vi "Write Ext.vi"(8 "Error In":errorcluster) -> (0 "Error Out":errorcluster)   [LabVIEW 2017, in "Tests.lvlib" / "Writer.lvlib"]
uses:
  Writer.lvlib
  src/LabPack/Public/Writer/Private/Write Ext by Value.vi
  <vilib>/addons/_JKI Toolkits/Caraya/classes/Test/Test.lvclass
  <vilib>/addons/_JKI Toolkits/Caraya/classes/Assert/Assert.lvclass
  src/LabPack/Public/Writer/Writer.lvclass
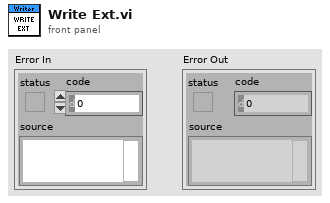
[diagram p1: front panel]
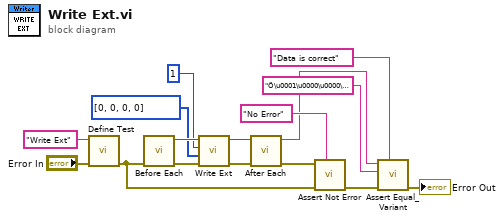
[diagram p0: block diagram]
diagram:
  n1 = call <vilib>:"Define Test.vi"("error in (no error)"="Error In", "Label (VI Title)"="Write Ext") -> ("error out"=w12:errorcluster)  [unwired: 9 in]
  n2 = call "Before Each.vi"("Error In"=w12) -> ("Error Out"=w8:errorcluster, "Writer Out"=w7:refnum<class "Writer.lvclass">)  [unwired: 9 in]
  n3 = call-poly "Write Ext.vi"("Error In"=w8, "Data"=u8[] [0, 0, 0, 0] ("Value"), "Type"=i8 1, "Writer In"=w7) -> ("Error Out"=w5:errorcluster, "Writer Out"=w6:refnum<class "Writer.lvclass">)  [unwired: 6 in]
  n4 = call "After Each.vi"("Error In"=w5, "Writer In"=w6) -> ("Error Out"=w11:errorcluster, "Data"=w4:string)  [unwired: 8 in]
  n5 = call <vilib>:"Assert Not Error.vi"("Label"="No Error", "error in (no error)"=w12, "Not Error?"=w11) -> ("error out"=w14:errorcluster)  [unwired: 8 in]
  n6 = call <vilib>:"Assert Equal_Variant.vi"("Label"="Data is correct", "error in (no error)"=w14, "Y"="Ö\u0001\u0000\u0000\u0000\u0000" ("Data"), "X"=w4) -> ("error out"=→"Error Out":errorcluster)  [unwired: 7 in]
